vi "arm pid.vi"(1 "Setpoint":dbl, 2 "Autotune?":bool) -> (0 "Output":dbl)   [LabVIEW 2013]
uses:
  UberCode Suffield Philification/typedefs/DevRef Type.ctl
  typedefs/fg_typedef.ctl
  <vilib>/addons/control/pid/pid.llb/PID (DBL).vi
  <vilib>/addons/control/pid/NI_PID_autopid.lvlib
  <vilib>/addons/control/pid/NI_PID_pid.lvlib
panel:
  in  "autotuning parameters":T1={"controller type"=1, "relay cycles"=3, "relay amplitude"=1.0, "control specification"=2, "PV noise level"=0.1} {"controller type" items=["PID", "PI", "P"]; "control specification" items=["normal", "fast", "slow"]}
  # "Things needing Tuning"
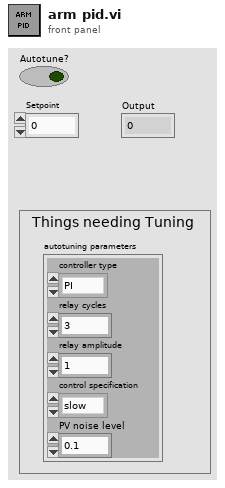
[diagram p1: front panel]
types:
  T1 = cluster{"controller type":u16, "relay cycles":i32, "relay amplitude":dbl, "control specification":u16, "PV noise level":dbl}
  T2 = typedef "fg_typedef.ctl" = enum16{"Get", "Set"}
  T3 = typedef "DevRef Type.ctl" = enum16{"Shooter Solenoid", "Latch Solenoid", "Right Up Sensor", "Right Down Sensor", "Hold Sensor", "Arm Encoder"}
  T4 = cluster{"proportional gain (Kc)":dbl, "integral time (Ti, min)":dbl, "derivative time (Td, min)":dbl}
  T5 = typedef "WPI_EncoderDevRef.ctl" = cluster{"DevStatus":errorcluster, "EncoderIndex":T6, "CounterIndex":T7, "DistancePerCount":dbl, "Decoding Type":T8}
  T6 = typedef "FPGA_EncoderIdx.ctl" = enum8{"Enc 0", "Enc 1", "Enc 2", "Enc 3", "Invalid"}
  T7 = typedef "FPGA_CounterCtrSystemIndex.ctl" = enum8{"Ctr 0", "Ctr 1", "Ctr 2", "Ctr 3", "Ctr 4", "Ctr 5", "Ctr 6", "Ctr 7", "Invalid"}
  T8 = typedef "WPI_EncoderType.ctl" = enum16{"1x", "2x", "4x"}
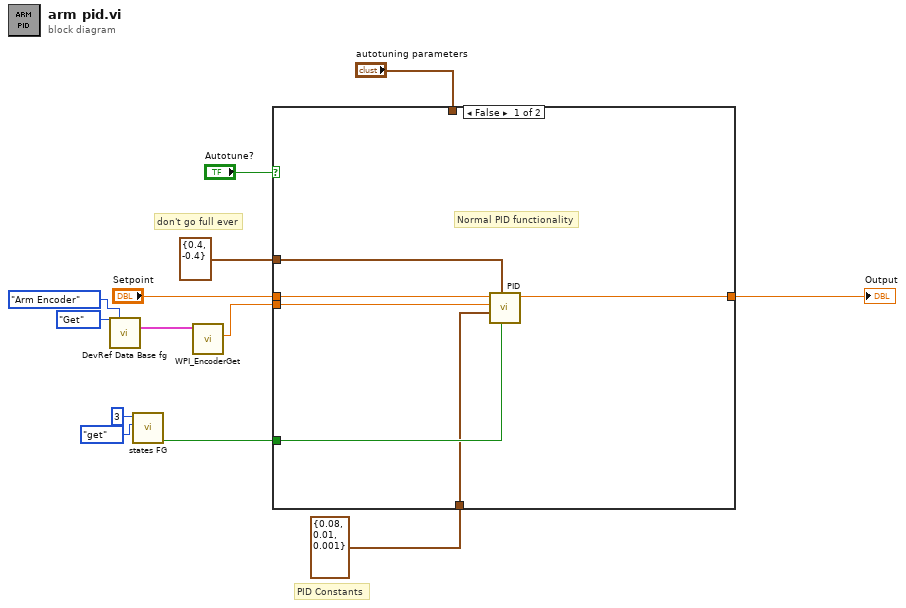
[diagram p0: block diagram]
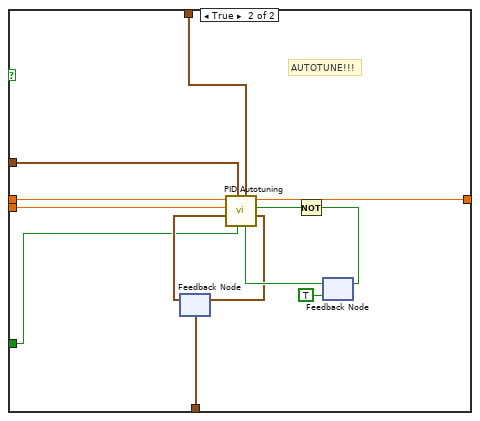
[diagram p2: hidden frame]
diagram:
  # "don't go full ever"
  # "PID Constants"
  n1 = call "DevRef Data Base fg.vi"("Menu"=fg_typedef."Get", "DevRef to Get"=DevRef_Type."Arm Encoder") -> ("Selected Encoder"=w4:T5)  [unwired: 23 in, 2 out]
  n2 = call "states FG.vi"("menu (get)"=enum16{"set", "get"}."get", "Loop ID"=3) -> ("first call?"=w8:bool)  [unwired: 6 in, 3 out]
  n3 = call <vilib>:"WPI_EncoderGet.vi"("EncoderDevRef"=w4) -> ("Distance"=w11:dbl)  [unwired: 5 in, 5 out]
  n4 = case shown="False" "Autotune?" {
    tunnel: "Setpoint" -> [w19 w32]
    tunnel: [w18 w31] -> w12
    tunnel: w11 -> [w16 w24]
    tunnel: w8 -> [w17 w23]
    tunnel: T4 {"proportional gain (Kc)"=0.08, "integral time (Ti, min)"=0.01, "derivative time (Td, min)"=0.001} ("PID gains") -> [w15 w22]
    tunnel: cluster{"output high":dbl, "output low":dbl} {"output high"=0.4, "output low"=-0.4} ("output range") -> [w14 w21]
    tunnel: "autotuning parameters" -> [_ w20]
    frame False {
      # "Normal PID functionality"
      n5 = call-poly <vilib>:"PID.vi"("reinitialize? (F)"=w17, "output range"=w14, "PID gains"=w15, "process variable"=w16, "setpoint"=w19) -> ("output"=w18:dbl)  [unwired: 5 in, 1 out]
    }
    frame True {
      # "AUTOTUNE!!!"
      n6 = feedback #1(w22) -> (w25:T4)
      n7 = feedback #2(TRUE) -> (w28:bool)
      n8 = call <vilib>:"PID Autotuning.vi"("autotune? (F)"=w28, "autotuning parameters"=w20, "reinitialize? (F)"=w23, "output range"=w21, "PID gains"=w25, "process variable"=w24, "setpoint"=w32) -> ("PID gains out"=w26:T4, "tuning completed?"=w30:bool, "output"=w31:dbl)  [unwired: 1 in, 1 out]
      n9 = feedback-in #1(w26) -> ()
      n10 = Not(x=w30) -> (.not. x?=w29:bool)
      n11 = feedback-in #2(w29) -> ()
    }
  }
  "Output" <- w12
